vi "Pkt - Get Controller Name.vi"(8 "error in (no error)":errorcluster, 11 "Packet Ref In":T1=18446744073709551615 format="%.0x") -> (0 "error out":errorcluster, 2 "Name":string, 3 "Packet Ref out":T1=18446744073709551615 format="%.0x")   [LabVIEW 2019, in "UDP-Custom-Device System Explorer.lvlib"]
uses:
  UDP-Custom-Device System Explorer.lvlib
  <vilib>/NI VeriStand/Custom Device API/Custom Device Item Ref.ctl
  NationalInstruments.VeriStand.SystemDefinitionAPI
  <vilib>/NI VeriStand/Custom Device Offline API/Custom Device Offline API.lvlib
  <vilib>/NI VeriStand/Custom Device Tools/Custom Device Utility Library/Custom Device Utility Library.lvlib
  <vilib>/NI VeriStand/Custom Device API/Custom Device API.lvlib
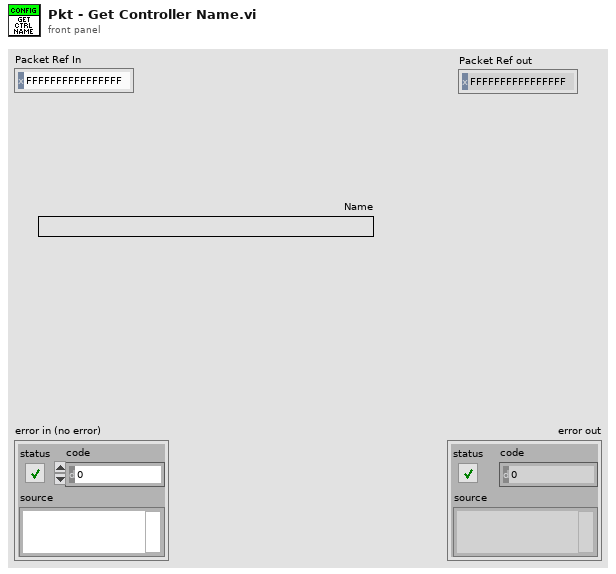
[diagram p1: front panel]
types:
  T1 = typedef "Custom Device API.lvlib/Custom Device Item Ref.ctl" = u64
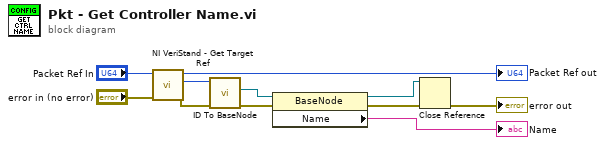
[diagram p0: block diagram]
diagram:
  n1 = call <vilib>:"NI VeriStand - Get Target Ref.vi"("error in"="error in (no error)", "Item Ref in"="Packet Ref In") -> ("error out"=w8:errorcluster, "Target Ref"=w9:T1, "Item Ref out"=→"Packet Ref out":T1)  [unwired: 6 in, 1 out]
  n2 = call <vilib>:"ID To BaseNode.vi"("error in (no error)"=w8, "ID in"=w9) -> ("error out"=w6:errorcluster, "BaseNode"=w7:refnum<k24>)  [unwired: 7 in, 1 out]
  n3 = property class="BaseNode"(reference=w7, error in=w6) -> (reference out=w3:refnum<k24>, error out=w2:errorcluster, "Name"=→"Name":string)
  n4 = Close Reference(reference=w3, error in (no error)=w2) -> (error out=→"error out":errorcluster)
